vi "Rising Edge Detect.vi"(7 "Reset?":bool, 11 "Boolean":bool) -> (3 "Rising Edge?":bool)   [LabVIEW 2021]
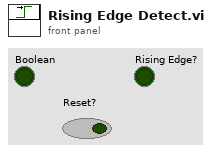
[diagram p1: front panel]
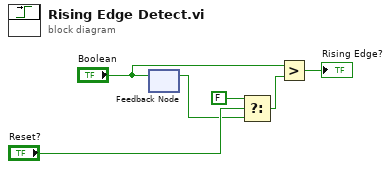
[diagram p0: block diagram]
diagram:
  n1 = feedback-in #1("Boolean") -> ()
  n2 = feedback #1() -> (w3:bool)  [unwired: 1 in]
  n3 = Select(t=FALSE, s="Reset?", f=w3) -> (s? t:f=w2:bool)
  n4 = Greater?(x="Boolean", y=w2) -> (0:→"Rising Edge?":bool)
